vi "Write Power FIFO Direct Dispatch.vi"(6 "FIFO Timestamps":T1, 8 "error in (no error)":errorcluster, 9 "Timeout (ms)":i32=100, 10 "Data In":T2[](array[typedef])=[{"measurement"=[], "dT"=0.0, "Timestamp"=0, "Read Lock"=FALSE}, {"measurement"=[], "dT"=0.0, "Timestamp"=0, "Read Lock"=FALSE}], 11 "CIFTag in":refnum<class "CIFChannels.lvclass">) -> (0 "error out":errorcluster, 1 "timed out?":bool, 2 "Data Out":T2[](array[typedef]), 3 "CIFTag out":refnum<class "CIF_NIChn_Fifo_Power.lvclass">)   [LabVIEW 2021, in "CIF_NIChn_Fifo_Power.lvclass"]
uses:
  CIF_NIChn_Fifo_Power.lvclass
  CIF_NIChn_Fifo_Power.lvclass/CIF_NIChn_Fifo_Power.ctl
  NIChn/CIF_NIChn.lvclass
  <vilib>/CIFChannels/CIFChannelCore.lvlib
  D:/dev/CIF-LVCore/src/Channels/CIF_NIChn/NIChn/CIF_NIChn.lvclass
  D:/dev/CIF-LVCore/src/Channels/CIFChannels/CIFChannels.lvclass
  D:/dev/CIF-LVCore/src/Channels/CIF_NIChn/FIFO_Power/CIF_NIChn_Fifo_Power.lvclass
  CIFChannels/CIFChannels.lvclass
  ChannelCommon/typedef/Datatype Waveform.ctl
  ChannelCommon/ChannelCommon.lvlib
  ChannelCommon/typedef/TimeStamps.ctl
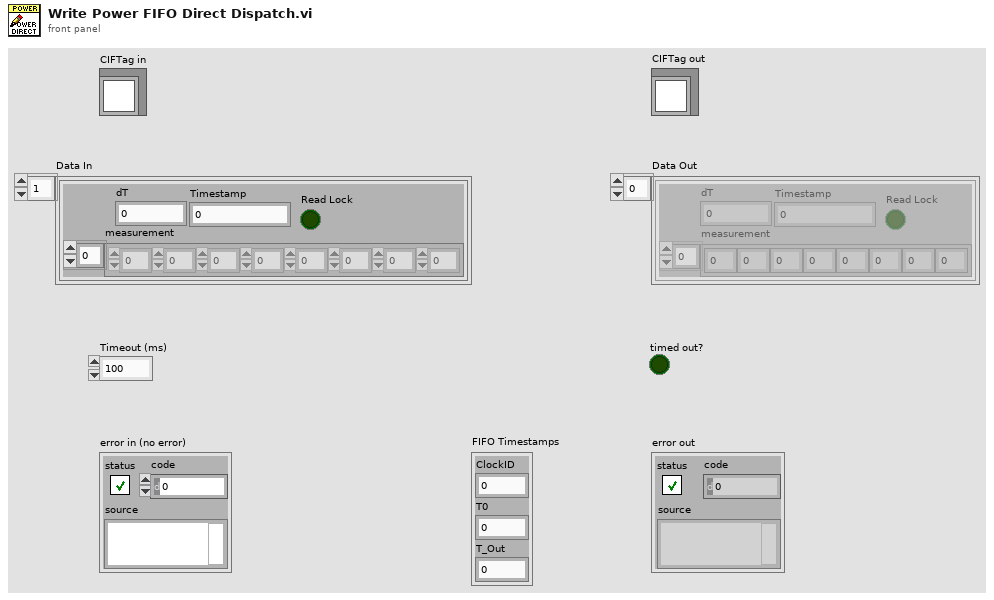
[diagram p1: front panel]
types:
  T1 = typedef "ChannelCommon.lvlib/TimeStamps.ctl" = cluster{"ClockID":u8, "T0":i64, "T_Out":i64}
  T2 = typedef "ChannelCommon.lvlib/Datatype Waveform.ctl" = cluster{"measurement":dbl[], "dT":dbl, "Timestamp":i64, "Read Lock":bool}
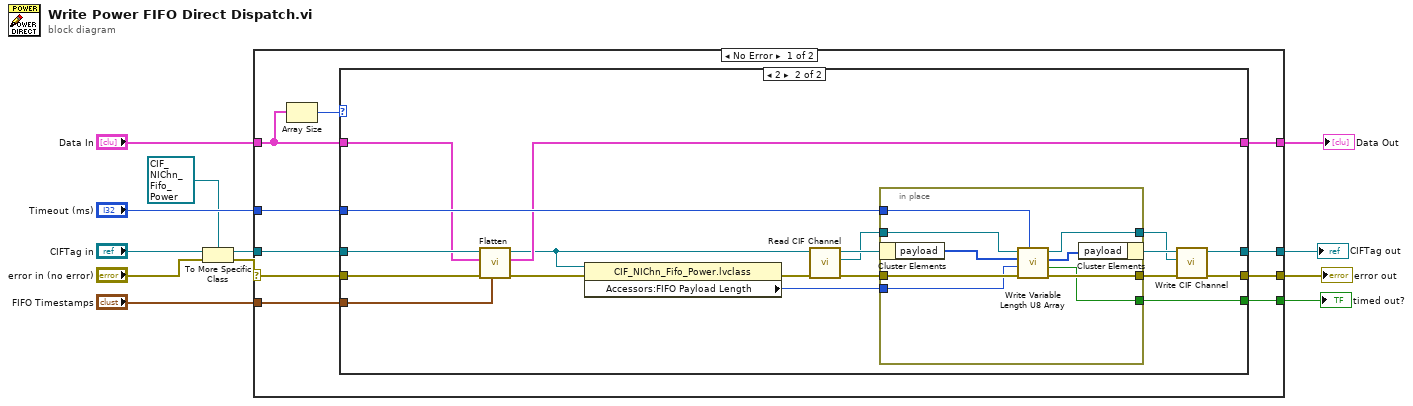
[diagram p0: block diagram]
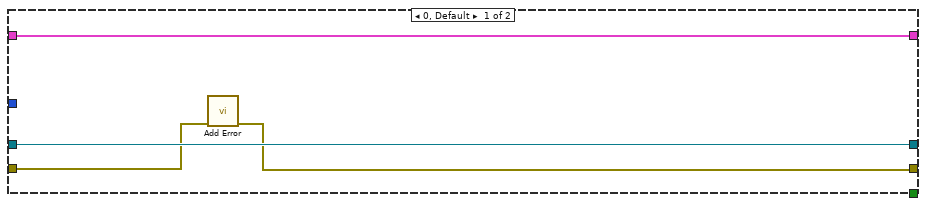
[diagram p2: hidden frame]
diagram:
  n1 = To More Specific Class(target class=refnum<class "CIF_NIChn_Fifo_Power.lvclass"> refnum ("CIFTag in"), reference="CIFTag in", error in="error in (no error)") -> (specific class reference=w6:refnum<class "CIF_NIChn_Fifo_Power.lvclass">, error out=w4:errorcluster)
  n2 = case shown="No Error" w4 {
    selector: w4 -> [w17 w57]
    tunnel: [w19 w57] -> w12
    tunnel: [w21 w56] -> w11
    tunnel: w6 -> [w18 w56]
    tunnel: [w22 _] -> w10
    tunnel: "Timeout (ms)" -> [w20 _]
    tunnel: "Data In" -> [w14 w55]
    tunnel: [w16 w55] -> w2
    tunnel: "FIFO Timestamps" -> [w13 _]
    frame No Error {
      n3 = Array Size(array=w14) -> (size(s)=w15:i32)
      n4 = case shown="2" w15 {
        tunnel: [_ w45] -> w22
        tunnel: [w25 w41] -> w21
        tunnel: w20 -> [_ w37]
        tunnel: [w23 w36] -> w19
        tunnel: w18 -> [w25 w34]
        tunnel: w17 -> [w24 w32]
        tunnel: w14 -> [w26 w30]
        tunnel: [w26 w29] -> w16
        tunnel: w13 -> [_ w28]
        frame 0, Default {
          n5 = call "Add Error.vi"("error in (no error)"=w24) -> ("error out"=w23:errorcluster)  [unwired: 10 in]
        }
        frame 2 {
          n6 = call "Flatten.vi"("FIFO Timestamps"=w28, "error in (no error)"=w32, "Data"=w30, "CIFTag in"=w34) -> ("error out"=w33:errorcluster, "Data out"=w29:T2[], "CIFTag out"=w27:refnum<class "CIF_NIChn_Fifo_Power.lvclass">)  [unwired: 5 in]
          n7 = property class="CIF_NIChn_Fifo_Power.lvclass"(reference=w27, error in=w33) -> (error out=w35:errorcluster, "Accessors:FIFO Payload Length"=w31:u64)  [unwired: 1 out]
          n8 = call "Read CIF Channel.vi"("error in (no error)"=w35, "CIFTag in"=w27) -> ("error out"=w43:errorcluster, "CIF Channel"=w39:refnum<k21>, "CIFTag out"=w44:refnum<class "CIF_NIChn_Fifo_Power.lvclass">)  [unwired: 7 in]
          n9 = in-place {
            in-place-border: w43 -> [w54]
            in-place-border: [w53] -> w40
            in-place-border: [w52] -> w45
            in-place-border: w39 -> [w51]
            in-place-border: [w50] -> w38
            in-place-border: w37 -> [w49]
            in-place-border: w31 -> [w47]
            n10 = in-place-cluster #1(w44) -> ("payload"=w48:u8[])
            n11 = call <vilib>:"Write Variable Length U8 Array.vi"("Timeout (ms)"=w49, "error in"=w54, "numElements"=w47, "U8 Array in"=w48, "CIF Channel in"=w51) -> ("error out"=w53:errorcluster, "Timed out?"=w52:bool, "U8 Array out"=w46:u8[], "CIF Channel out"=w50:refnum<k21>)  [unwired: 3 in]
            n12 = in-place-cluster #1("payload"=w46) -> (w42:refnum<class "CIF_NIChn_Fifo_Power.lvclass">)
          }
          n13 = call "Write CIF Channel.vi"("error in (no error)"=w40, "CIF Channel"=w38, "CIFTag in"=w42) -> ("error out"=w36:errorcluster, "CIFTag out"=w41:refnum<class "CIF_NIChn_Fifo_Power.lvclass">)  [unwired: 7 in]
        }
      }
    }
    frame Error {
    }
  }
  "error out" <- w12
  "CIFTag out" <- w11
  "timed out?" <- w10
  "Data Out" <- w2
